vi "Adjust Bit Depth x8 (SubVI).vi"(0 "Minimum":u8, 2 "Bit Depth":u8, 5 "Stat. Valid?":bool, 11 "Pixel Data":u64, 12 "Block Size x2":u16, 13 "Pixel Valid?":bool) -> (14 "Output Valid?":bool, 16 "Data Out":T1, 19 "Bid Depth Out":u8)   [LabVIEW 2015]
uses:
  Controls (FPGA)/Sync Block Statistics.ctl
  <vilib>/rvi/DataTransferAndStorage/Container/Common/niFpgaContainerGetUniqueNameForEmu.vi
  <vilib>/rvi/DataTransferAndStorage/Container/Common/niFpgaContainerSetEmuInfo.vi
  <vilib>/rvi/eio/common/nirviEmuReportErrorAndStop.vi
  <vilib>/rvi/Emulation/niFpgaEmulationIsFPGAContextNoSignature.vi
  <vilib>/rvi/Emulation/niFpgaSctlEmulationGetInTimedLoop.vi
  <vilib>/rvi/errors/niFpgaSetErrorForExecOnDevCompSimple.vi
  <vilib>/rvi/FIFO/Fifo_Resource/nirvififoEmulationSetSize.vi
  <vilib>/rvi/FIFO/Fifo_Resource/nirviFifoEmulationQueueMgr.vi
  <instcachedir>/0/nirviFifoEmulationQueueMgr_E5CAEC123FF24DC58D834DCA3CDAA9B5.lvgen/nirviFifoEmulationQueueMgr_E5CAEC123FF24DC58D834DCA3CDAA9B5_007.vi
  <vilib>/rvi/FIFO/Fifo_Resource/nirvififoEmulationDetermineInputValidOut.vi
  <vilib>/rvi/FIFO/Fifo_Resource/nirvififoEmulationCreateLock.vi
  <vilib>/rvi/Emulation/niFpgaProcessEmulError.vi
  <vilib>/rvi/FIFO/Fifo_Resource/nirvififoEmulationObtainLock.vi
  <vilib>/rvi/FIFO/Fifo_Resource/nirvififoEmulationReleaseLock.vi
  <vilib>/rvi/occurrence/nirviWaitOnOccurrenceBase.vi
  <vilib>/rvi/errors/nirviReportUnexpectedCaseInternalError.vi
  <vilib>/rvi/errors/nirviReportUnexpectedCaseInternalError (U32).vi
  <instcachedir>/0/nirviFifoEmulationQueueMgr_E5CAEC123FF24DC58D834DCA3CDAA9B5.lvgen/nirviFifoEmulationQueueMgr_E5CAEC123FF24DC58D834DCA3CDAA9B5_004.vi
  <vilib>/Utility/error.llb/Clear Errors.vi
  <vilib>/rvi/LocalResourceManager/LocalResourceManager.xnode
  <vilib>/rvi/DataTransferAndStorage/Container/XNode/niFpgaContainer.xnode
  <vilib>/rvi/FIFO/Fifo_Resource/nirvififoEmulationWrite.vi
  <vilib>/rvi/FIFO/Fifo_Resource/nirvififoEmulationRead.vi
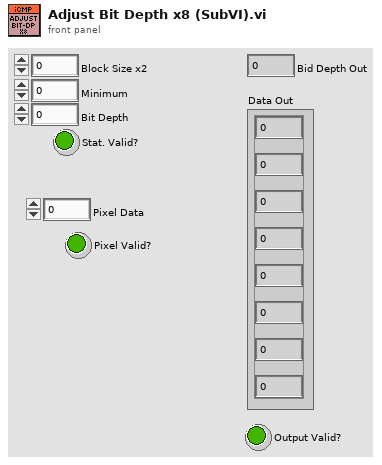
[diagram p1: front panel]
types:
  T1 = cluster{"Numeric Control":u8, "Numeric Control":u8, "Numeric Control":u8, "Numeric Control":u8, "Numeric Control":u8, "Numeric Control":u8, "Numeric Control":u8, "Numeric Control":u8}
  T2 = typedef "Sync Block Statistics.ctl" = enum16{"Wait for Start", "Wait for End"}
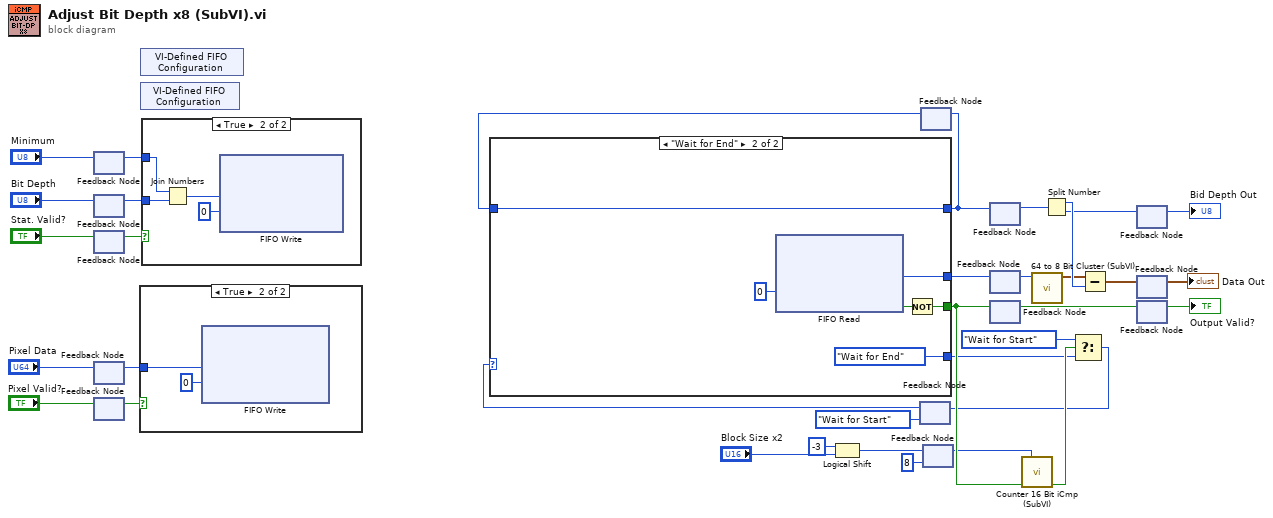
[diagram p0: block diagram]
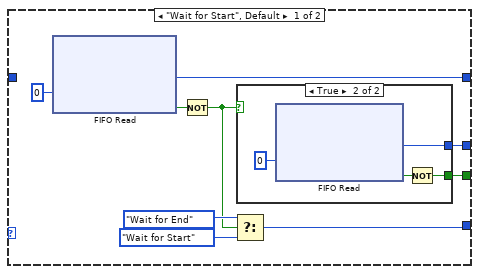
[diagram p2: hidden frame]
diagram:
  n1 = feedback-in #1("Minimum") -> ()
  n2 = feedback #1() -> (w12:u8)  [unwired: 1 in]
  n3 = feedback-in #2("Bit Depth") -> ()
  n4 = feedback #2() -> (w11:u8)  [unwired: 1 in]
  n5 = feedback-in #3("Stat. Valid?") -> ()
  n6 = feedback #3() -> (w10:bool)  [unwired: 1 in]
  n7 = feedback-in #4("Pixel Data") -> ()
  n8 = feedback #4() -> (w9:u64)  [unwired: 1 in]
  n9 = feedback-in #5("Pixel Valid?") -> ()
  n10 = feedback #5() -> (w8:bool)  [unwired: 1 in]
  n11 = case shown="True" w8 {
    tunnel: w9 -> [_ w36]
    frame False {
    }
    frame True {
      n12 = xnode ("FIFO Write")("Element"=w36, "Timeout"=0) -> ()  [unwired: 1 in, 2 out]
    }
  }
  n13 = xnode "VI-Defined FIFO Configuration"() -> ()  [unwired: 1 out]
  n14 = xnode "VI-Defined FIFO Configuration"() -> ()  [unwired: 1 out]
  n15 = case shown="True" w10 {
    tunnel: w12 -> [_ w39]
    tunnel: w11 -> [_ w38]
    frame False {
    }
    frame True {
      n16 = Join Numbers(hi=w39, lo=w38) -> ((hi.lo)=w40:u16)
      n17 = xnode ("FIFO Write")("Element"=w40, "Timeout"=0) -> ()  [unwired: 1 in, 2 out]
    }
  }
  n18 = Logical Shift(y=i16 -3, x="Block Size x2") -> (x << y=w4:u16)
  n19 = feedback #6(Sync_Block_Statistics."Wait for Start" ("Sync Block Statistics")) -> (w30:T2)
  n20 = feedback #7() -> (w28:u16)  [unwired: 1 in]
  n21 = case shown="\"Wait for End\"" w30 {
    tunnel: [w48 Sync_Block_Statistics."Wait for End" ("Sync Block Statistics")] -> w23
    tunnel: [w45 w55] -> w27
    tunnel: [w43 w59] -> w21
    tunnel: w28 -> [_ w59]
    tunnel: [w42 w56] -> w20
    frame "Wait for Start", Default {
      n22 = xnode ("FIFO Read")("Timeout"=0) -> ("Element"=w43:u16, "Timed Out?"=w46:bool)  [unwired: 1 in, 1 out]
      n23 = Not(x=w46) -> (.not. x?=w44:bool)
      n24 = Select(t=Sync_Block_Statistics."Wait for End" ("Sync Block Statistics"), s=w44, f=Sync_Block_Statistics."Wait for Start" ("Sync Block Statistics")) -> (s? t:f=w48:T2)
      n25 = case shown="True" w44 {
        tunnel: [_ w52] -> w45
        tunnel: [_ w51] -> w42
        frame False {
        }
        frame True {
          n26 = xnode ("FIFO Read")("Timeout"=0) -> ("Element"=w51:u64, "Timed Out?"=w53:bool)  [unwired: 1 in, 1 out]
          n27 = Not(x=w53) -> (.not. x?=w52:bool)
        }
      }
    }
    frame "Wait for End" {
      n28 = xnode ("FIFO Read")("Timeout"=0) -> ("Element"=w56:u64, "Timed Out?"=w58:bool)  [unwired: 1 in, 1 out]
      n29 = Not(x=w58) -> (.not. x?=w55:bool)
    }
  }
  n30 = feedback-in #7(w21) -> ()
  n31 = feedback-in #8(w4) -> ()
  n32 = feedback #8(u16 8) -> (w2:u16)
  n33 = feedback-in #9(w21) -> ()
  n34 = feedback #9() -> (w16:u16)  [unwired: 1 in]
  n35 = feedback-in #10(w20) -> ()
  n36 = feedback #10() -> (w7:u64)  [unwired: 1 in]
  n37 = feedback-in #11(w27) -> ()
  n38 = feedback #11() -> (w15:bool)  [unwired: 1 in]
  n39 = call "Counter 16 Bit iCmp (SubVI).vi"("Max. Count"=w2, "Enable"=w27) -> ("Count End?"=w24:bool)  [unwired: 11 in, 2 out]
  n40 = call "64 to 8 Bit Cluster (SubVI).vi"("Data In"=w7) -> ("Data Out"=w6:T1)  [unwired: 10 in]
  n41 = Split Number(x=w16) -> (hi(x)=w19:u8, lo(x)=w18:u8)
  n42 = Select(t=Sync_Block_Statistics."Wait for Start" ("Sync Block Statistics"), s=w24, f=w23) -> (s? t:f=w22:T2)
  n43 = feedback-in #6(w22) -> ()
  n44 = Subtract(x=w6, y=w19) -> (x-y=w17:T1)
  n45 = feedback-in #12(w18) -> ()
  n46 = feedback #12() -> (→"Bid Depth Out":u8)  [unwired: 1 in]
  n47 = feedback-in #13(w17) -> ()
  n48 = feedback #13() -> (→"Data Out":T1)  [unwired: 1 in]
  n49 = feedback-in #14(w15) -> ()
  n50 = feedback #14() -> (→"Output Valid?":bool)  [unwired: 1 in]
